vi "HP81110A Query Trigger Source.vi"(8 "error in (no error)":errorcluster, 11 "VISA session":refnum<visa-resource-name>) -> (0 "error out":errorcluster, 2 "Trigger (Bit Period) Source (0:Internal PLL)":T1(ring)=enum."Clock Input", 3 "dup VISA session":refnum<visa-resource-name>)   [LabVIEW 2009]
doc: "This VI queries the trigger (bit period) source. Results can be: \n0 = Immediate (internal oscillator)\n1 = Internal PLL\n2 = Clock Input"
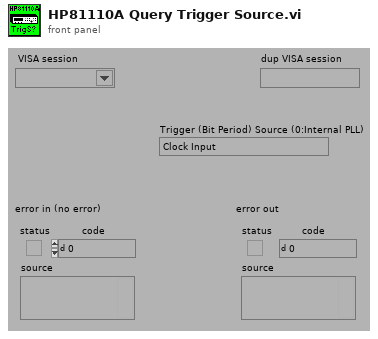
[diagram p1: front panel]
types:
  T1 = enum16{"Immediate (via internal oscillator)", "Internal PLL", "Clock Input"}
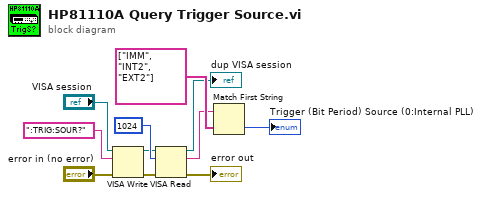
[diagram p0: block diagram]
diagram:
  n1 = VISA Write(VISA resource name="VISA session", write buffer=":TRIG:SOUR?", error in (no error)="error in (no error)") -> (VISA resource name out=w5:refnum<visa-resource-name>, error out=w6:errorcluster)  [unwired: 1 out]
  n2 = VISA Read(VISA resource name=w5, byte count=u32 1024 ("byte count (0)"), error in (no error)=w6) -> (VISA resource name out=→"dup VISA session":refnum<visa-resource-name>, read buffer=w7:string, error out=→"error out":errorcluster)  [unwired: 1 out]
  n3 = Match First String(2:string[] ["IMM", "INT2", "EXT2"] ("string array"), 3:w7) -> (0:→"Trigger (Bit Period) Source (0:Internal PLL)":i32)  [unwired: 1 out]
